vi "Stop Core.vi"(10 "final error code":i32, 11 "Logger in":refnum<class "Logger.lvclass">) -> (3 "Logger out":refnum<class "Logger.lvclass">)   [LabVIEW 2021, in "Logger.lvclass"]
doc: "(<B>Filename</B>: Actor Framework.lvlib:Actor.lvclass:Stop Core.vi)\n\nDefines what the actor does before it stops. Use the <B>final error code</B> input to determine whether the actor shut down in response to an error.\n\nBy default, this method does nothing. A descendant class may override it to define behavior, such as shutting down any processes the actor initiated in its override of the Actor Core method."
uses:
  Logger.lvclass
  Logger.lvclass/Logger.ctl
  NHMFL_Core/Libraries/File/File Class/File.lvclass/File.ctl
  Read File.lvclass.vi
  NHMFL_Core/Libraries/File/File Class/Read Is open.vi
  Write File.lvclass.vi
  NHMFL_Core/Libraries/File/File Class/File.lvclass
  <vilib>/ActorFramework/Actor/Actor.lvclass
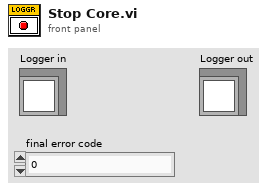
[diagram p1: front panel]
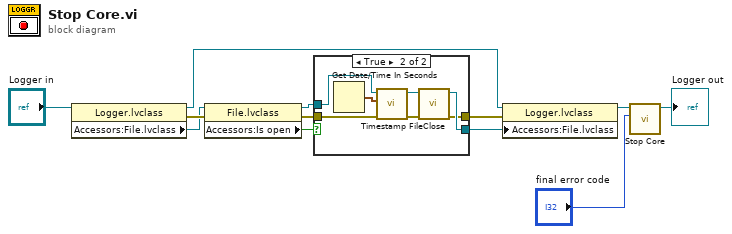
[diagram p0: block diagram]
diagram:
  n1 = property class="Logger.lvclass"(reference="Logger in") -> (reference out=w4:refnum<class "Logger.lvclass">, error out=w10:errorcluster, "Accessors:File.lvclass"=w7:refnum<class "File.lvclass">)  [unwired: 1 in]
  n2 = property class="File.lvclass"(reference=w7, error in=w10) -> (reference out=w6:refnum<class "File.lvclass">, error out=w8:errorcluster, "Accessors:Is open"=w5:bool)
  n3 = case shown="True" w5 {
    tunnel: w8 -> [w14 w17]
    tunnel: w6 -> [w13 w19]
    tunnel: [w13 w21] -> w3
    tunnel: [w14 w20] -> w2
    frame False {
    }
    frame True {
      n4 = Get Date/Time In Seconds() -> (seconds since 1Jan1904=w15:timestamp)
      n5 = call-dynamic "Timestamp File.vi"("error in (no error)"=w17, "Time Stamp"=w15, "File in"=w19) -> ("error out"=w16:errorcluster, "File out"=w18:refnum<class "File.lvclass">)  [unwired: 7 in]
      n6 = call-dynamic "Close.vi"("error in (no error)"=w16, "File in"=w18) -> ("error out"=w20:errorcluster, "File out"=w21:refnum<class "File.lvclass">)  [unwired: 6 in, 2 out]
    }
  }
  n7 = property class="Logger.lvclass"(reference=w4, error in=w2, "Accessors:File.lvclass"=w3) -> (reference out=w1:refnum<class "Logger.lvclass">)  [unwired: 1 out]
  n8 = call-parent "Stop Core.vi"("final error code"="final error code", "Actor in"=w1) -> ("Actor out"=→"Logger out":refnum<class "Logger.lvclass">)  [unwired: 9 in]
